vi "DQMH Stop Module.vi"(7 "Module Disk Path":path, 8 "error in (no error)":errorcluster, 11 "Application ref":refnum<vi>) -> (0 "error out":errorcluster)   [LabVIEW 2022 SP3, in "hse-dqmh-dynamicrequesters.lvlib"]
doc: "Calls the \"Stop Module\" request VI of the module in <b>Path to module directory</b>\n\n____\nHAMPEL SOFTWARE ENGINEERING v3.8.0 (2023-12-18 14:41)"
uses:
  hse-dqmh-dynamicrequesters.lvlib
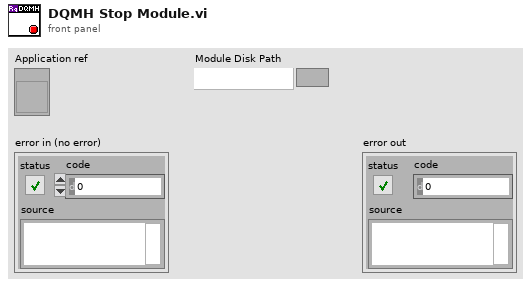
[diagram p1: front panel]
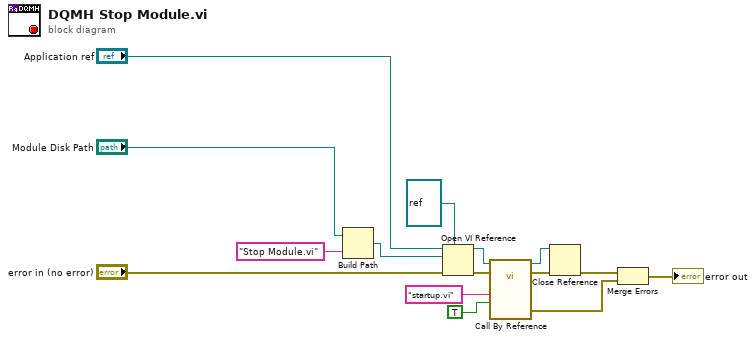
[diagram p0: block diagram]
diagram:
  n1 = Build Path(base path="Module Disk Path", name or relative path="Stop Module.vi") -> (appended path=w10:path)
  n2 = Open VI Reference(type specifier VI Refnum (for type only)=refnum<vi> refnum, application reference (local)="Application ref", vi path=w10, error in (no error)="error in (no error)") -> (vi reference=w9:refnum<vi>, error out=w7:errorcluster)  [unwired: 2 in]
  n3 = call-by-ref "?"(reference=w9, error in=w7, "Wait for Module to Stop? (F)"=TRUE, "Origin"="startup.vi") -> (reference out=w4:refnum<vi>, error out=w11:errorcluster, 0:"error out"=w12:errorcluster)  [unwired: 9 in]
  n4 = Close Reference(reference=w4, error in (no error)=w11) -> (error out=w5:errorcluster)
  n5 = Merge Errors(w5, w12) -> (→"error out":errorcluster)
